vi "GetColorFromStrCtrl.vi"(11 "str ref in":refnum<vi>) -> (2 "색 상자":u32(colorbox), 3 "str ref out":refnum<vi>)   [LabVIEW 2018, in "Library-Ctrl.lvlib"]
uses:
  Library-Ctrl.lvlib
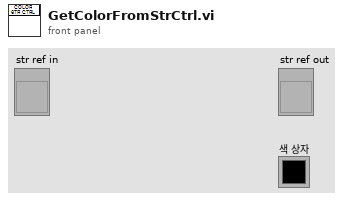
[diagram p1: front panel]
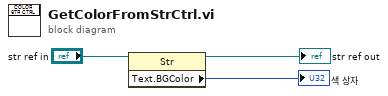
[diagram p0: block diagram]
diagram:
  n1 = property class="Str"(reference="str ref in") -> (reference out=→"str ref out":refnum<vi>, "Text.BGColor"=→"색 상자":u32)  [unwired: 1 in, 1 out]
